vi "exnSpectralBlock clear DDT y array.vi"(1 "Array In":waveform(dbl)[](array[waveform])) -> (0 "Array Out":waveform(dbl)[](array[waveform]))   [LabVIEW 2017]
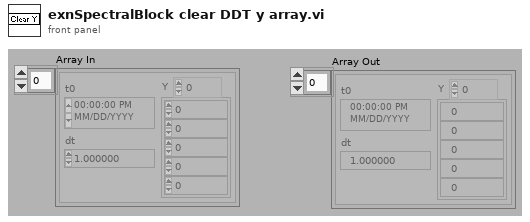
[diagram p1: front panel]
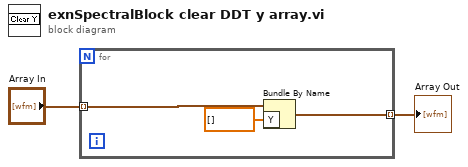
[diagram p0: block diagram]
diagram:
  n1 = for {
    tunnel: "Array In" -> [w5] mode=indexing
    tunnel: [w3] -> w1 mode=indexing
    n2 = Bundle By Name(cluster=w5, "Y"=dbl[] []) -> (w3:waveform(dbl))
  }
  "Array Out" <- w1
